vi "Execute.Initialize.vi"(8 "error in (no error)":errorcluster, 11 "State Variables":T1) -> (0 "error out":errorcluster, 3 "State Variables":T1)   [LabVIEW 2015]
uses:
  Types/Main.StateVariables.ctl
  <vilib>/Utility/miscctls.llb/LVPositionTypeDef.ctl
  Types/Execute.UserEventRefs.ctl
  <vilib>/NI Veristand/Execution/Workspace/SystemStateRegEventRef.ctl
  <vilib>/NI Veristand/Execution/Workspace/Target State Info.ctl
  <vilib>/NI Veristand/Execution/Workspace/Target State.ctl
  <vilib>/NI Veristand/Execution/WaveformStreaming/Waveform Data Watcher Event Data (DBL).ctl
  <vilib>/NI Veristand/Execution/WaveformStreaming/WaveformStreamSpecification.ctl
  NationalInstruments.VeriStand.ClientAPI
  <vilib>/NI Veristand/Execution/Workspace/SystemStateEventRef.ctl
  <vilib>/NI Veristand/Execution/Workspace/WorkspaceAPI.ctl
  Types/UI.Object.ctl
  Types/Waveforms.Info.ctl
  <vilib>/NI Veristand/Execution/WaveformStreaming/Registered Waveform Streams Data Event Refnum (DBL).ctl
  <vilib>/NI Veristand/Execution/WaveformStreaming/WaveformDataWatcherDBL.ctl
  <vilib>/NI Veristand/Execution/WaveformStreaming/WaveformStreamingAPI.ctl
  <vilib>/NI Veristand/Execution/Workspace/NI_VS Workspace ExecutionAPI.lvlib
  <vilib>/NI Veristand/Execution/WaveformStreaming/NI_VS Waveform Streaming Interface.lvlib
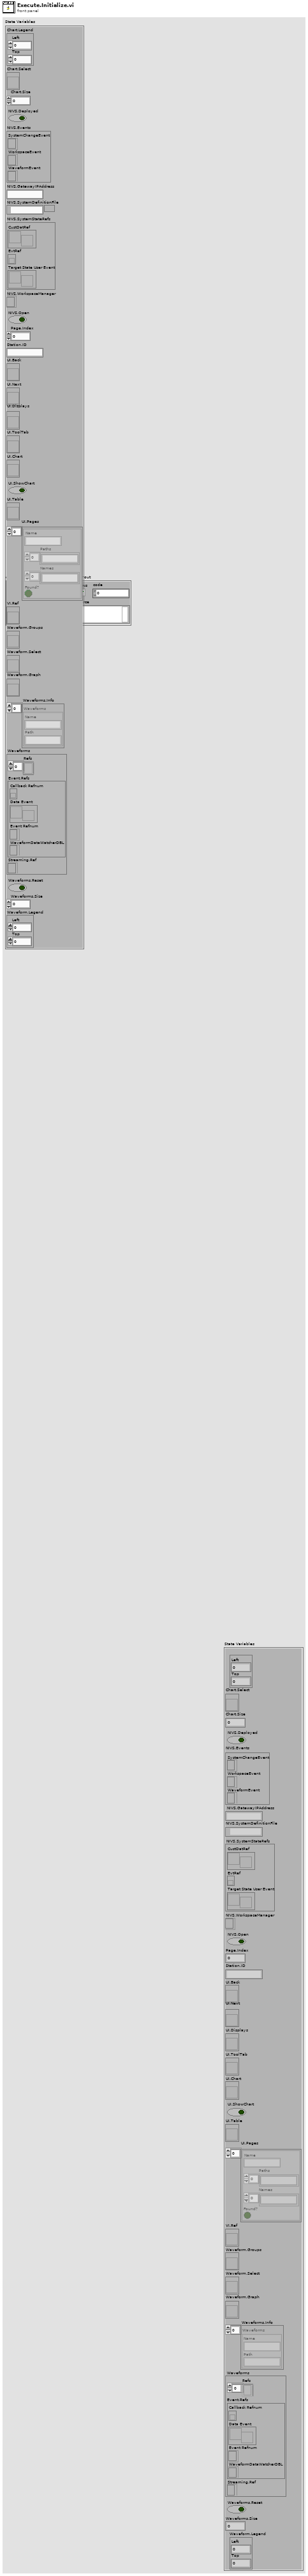
[diagram p1: front panel]
types:
  T1 = typedef "Main.StateVariables.ctl" = cluster{"Chart.Legend":T2, "Chart.Select":refnum<vi>, "Chart.Size":i32, "NIVS.Deployed":bool, "NIVS.Events":T3, "NIVS.GatewayIPAddress":string, "NIVS.SystemDefinitionFile":path, "NIVS.SystemStateRefs":T5, "NIVS.WorkspaceManager":T6, "NIVS.Open":bool, "Page.Index":u32, "Station.ID":string, "UI.Back":refnum<vi>, "UI.Next":refnum<vi>, "UI.Displays":refnum<vi>, "UI.ToolTab":refnum<vi>, "UI.Chart":refnum<vi>, "UI.ShowChart":bool, "UI.Table":refnum<vi>, "UI.Pages":T7[], "VI.Ref":refnum<vi>, "Waveform.Groups":refnum<vi>, "Waveform.Select":refnum<vi>, "Waveform.Graph":refnum<vi>, "Waveforms.Info":T8[], "Waveforms":cluster{"Refs":T9[], "Event.Refs":T10, "Streaming.Ref":T12}, "Waveforms.Reset":bool, "Waveforms.Size":i32, "Waveform.Legend":T2}
  T2 = typedef "LVPositionTypeDef.ctl" = cluster{"Left":i32, "Top":i32}
  T3 = typedef "Execute.UserEventRefs.ctl" = cluster{"SystemChangeEvent":T4, "WorkspaceEvent":refnum<event-registration>, "WaveformEvent":refnum<event-registration>}
  T4 = typedef "NI_VS Workspace ExecutionAPI.lvlib/SystemStateRegEventRef.ctl" = refnum<event-registration>
  T5 = typedef "NI_VS Workspace ExecutionAPI.lvlib/SystemStateEventRef.ctl" = cluster{"CustDatRef":refnum<user-event>, "EvtRef":refnum<k27>, "Target State User Event":refnum<user-event>}
  T6 = typedef "NI_VS Workspace ExecutionAPI.lvlib/WorkspaceAPI.ctl" = refnum<k24>
  T7 = typedef "UI.Object.ctl" = cluster{"Name":string, "Paths":string[], "Names":string[], "Found?":bool}
  T8 = typedef "Waveforms.Info.ctl" = cluster{"Name":string, "Path":string}
  T9 = typedef "NI_VS Waveform Streaming Interface.lvlib/WaveformStreamSpecification.ctl" = refnum<k24>
  T10 = typedef "NI_VS Waveform Streaming Interface.lvlib/Registered Waveform Streams Data Event Refnum (DBL).ctl" = cluster{"Callback Refnum":refnum<k27>, "Data Event":refnum<user-event>, "Event Refnum":refnum<event-registration>, "WaveformDataWatcherDBL":T11}
  T11 = typedef "NI_VS Waveform Streaming Interface.lvlib/WaveformDataWatcherDBL.ctl" = refnum<k24>
  T12 = typedef "NI_VS Waveform Streaming Interface.lvlib/WaveformStreamingAPI.ctl" = refnum<k24>
  T13 = enum8{"Enabled", "Disabled", "Disabled and Grayed Out"}
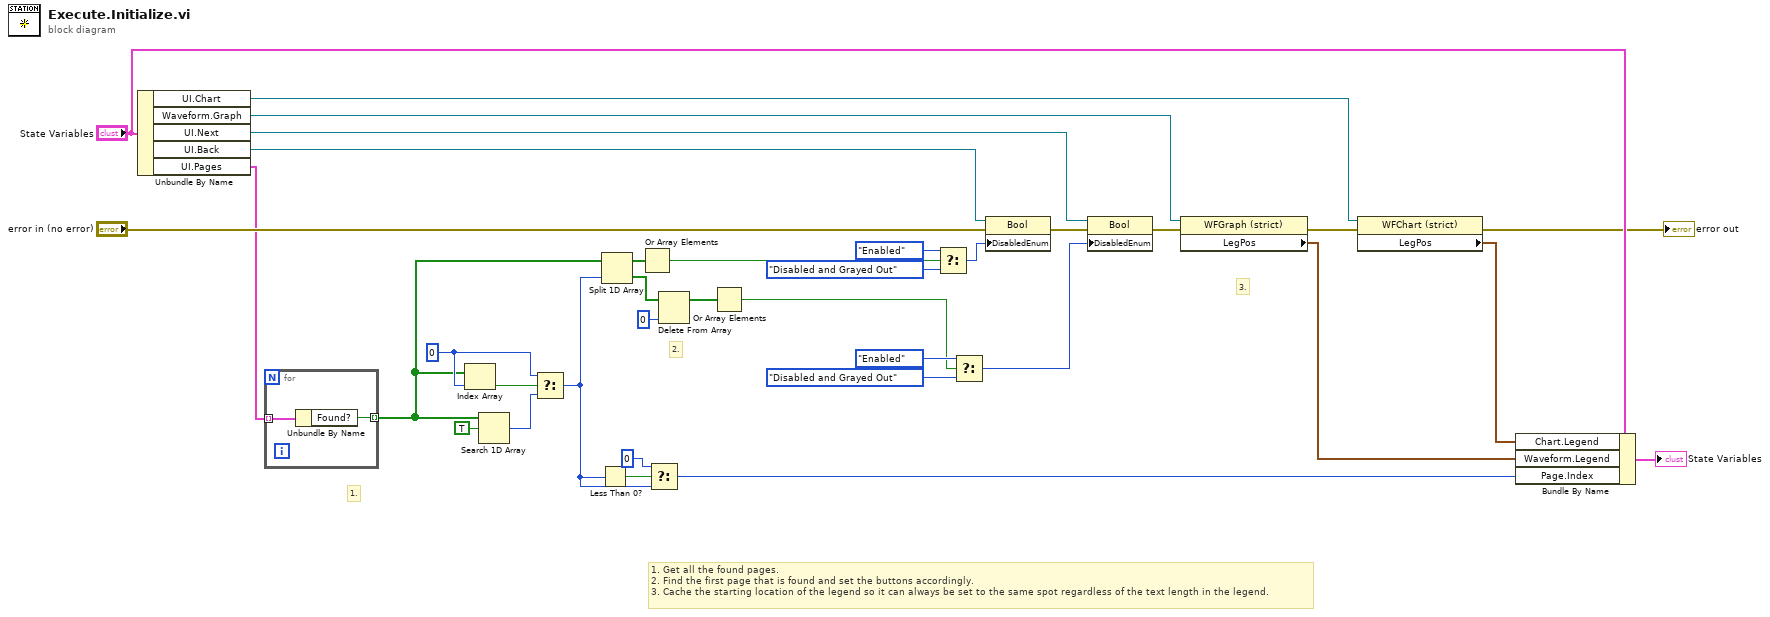
[diagram p0: block diagram]
diagram:
  w11 = 0
  # "1. Get all the found pages.\n2. Find the first page that is found and set the buttons accordingly.\n3. Cache the starting location of the legend so it can always be set to the same spot regardless of the text length in the legend."
  # "3."
  # "2."
  # "1."
  n1 = Unbundle By Name("State Variables") -> ("UI.Chart"=w4:refnum<vi>, "Waveform.Graph"=w26:refnum<vi>, "UI.Next"=w32:refnum<vi>, "UI.Back"=w33:refnum<vi>, "UI.Pages"=w10:T7[])
  n2 = for {
    tunnel: w10 -> [w37] mode=indexing
    tunnel: [w36] -> w9 mode=indexing
    n3 = Unbundle By Name(w37) -> ("Found?"=w36:bool)
  }
  n4 = Index Array(array=w9, index=w11) -> (element=w20:bool)
  n5 = Search 1D Array(1D array=w9, element=TRUE) -> (index of element=w19:i32)  [unwired: 1 in]
  n6 = Select(t=w11, s=w20, f=w19) -> (s? t:f=w7:i32)
  n7 = Less Than 0?(x=w7) -> (x < 0?=w8:bool)
  n8 = Split 1D Array(array=w9, index=w7) -> (first subarray=w18:bool[], second subarray=w16:bool[])
  n9 = Or Array Elements(Boolean array=w18) -> (logical OR=w17:bool)
  n10 = Select(t=u32 0, s=w8, f=w7) -> (s? t:f=w6:u32)
  n11 = Delete From Array(array=w16, index=0) -> (array with subset deleted=w14:bool[])  [unwired: 1 in, 1 out]
  n12 = Or Array Elements(Boolean array=w14) -> (logical OR=w13:bool)
  n13 = Select(t=T13."Enabled" ("Disabled"), s=w17, f=T13."Disabled and Grayed Out") -> (s? t:f=w27:T13)
  n14 = Select(t=T13."Enabled" ("Disabled"), s=w13, f=T13."Disabled and Grayed Out") -> (s? t:f=w28:T13)
  n15 = property class="Bool"(reference=w33, error in="error in (no error)", "DisabledEnum"=w27) -> (error out=w29:errorcluster)  [unwired: 1 out]
  n16 = property class="Bool"(reference=w32, error in=w29, "DisabledEnum"=w28) -> (error out=w25:errorcluster)  [unwired: 1 out]
  n17 = property class="WFGraph (strict)"(reference=w26, error in=w25) -> (error out=w3:errorcluster, "LegPos"=w22:T2)  [unwired: 1 out]
  n18 = property class="WFChart (strict)"(reference=w4, error in=w3) -> (error out=→"error out":errorcluster, "LegPos"=w1:T2)  [unwired: 1 out]
  n19 = Bundle By Name(cluster="State Variables", "Chart.Legend"=w1, "Waveform.Legend"=w22, "Page.Index"=w6) -> (→"State Variables":T1)
